vi "pyCode init.vi"(7 "pyCmdFilePath":path, 8 "error in (no error)":errorcluster, 10 "pyVersion":string, 11 "pyCode in":refnum<class "pyCode.lvclass">) -> (0 "error out":errorcluster, 3 "pyCode out":refnum<class "pyCode.lvclass">)   [LabVIEW 2018, in "pyCode.lvclass"]
uses:
  pyCode.lvclass
  pyCode.lvclass/pyCode.ctl
  Attributes/Write pyCmdFilePath.vi
  Attributes/Write pyCmdSession.vi
panel:
  out "standard output":string
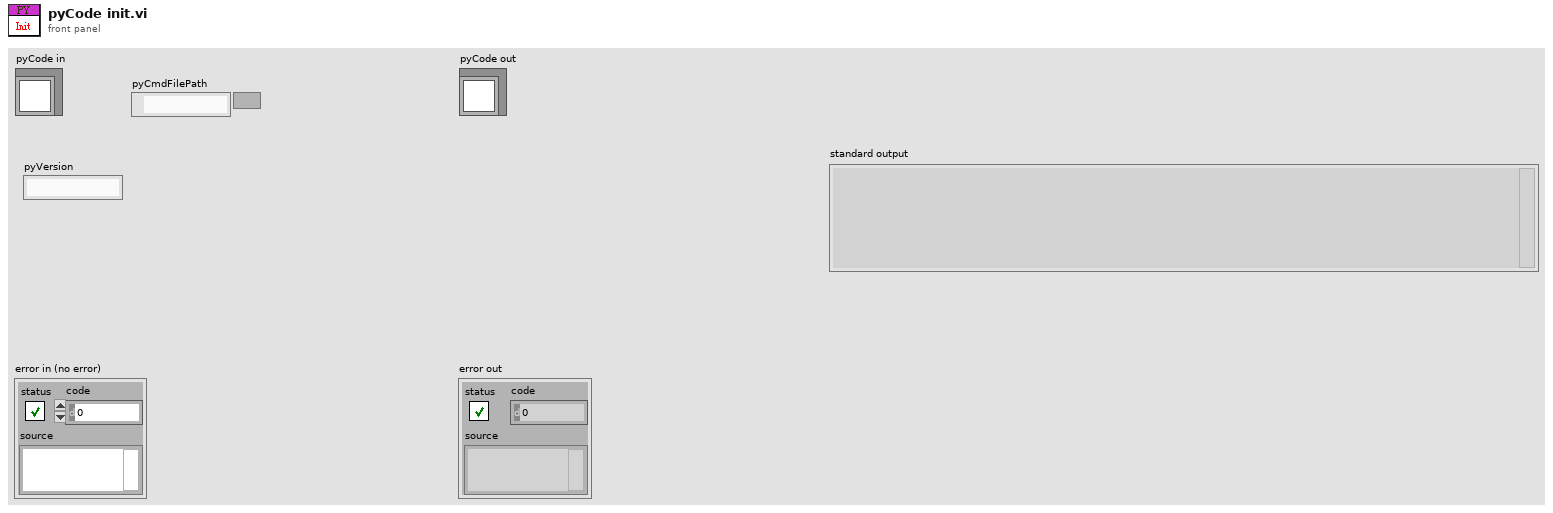
[diagram p1: front panel]
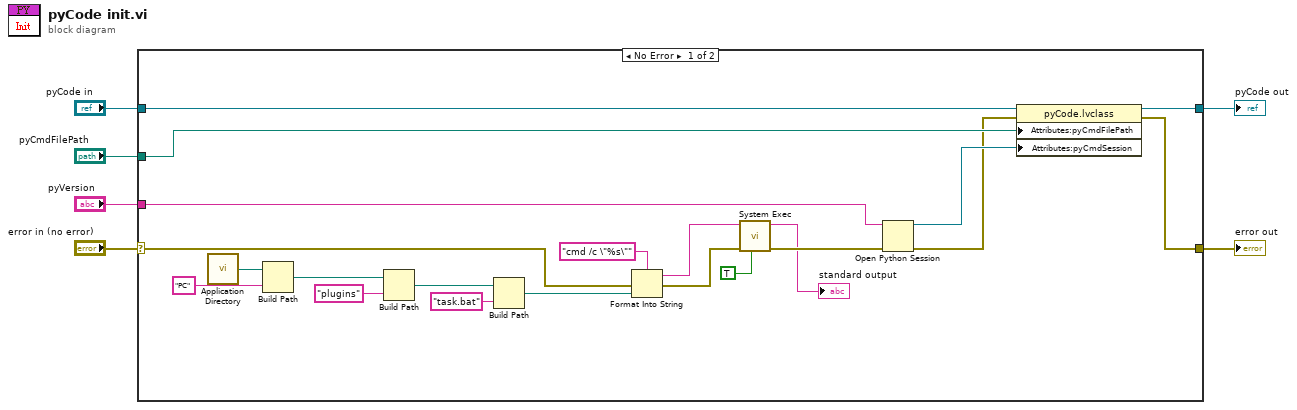
[diagram p0: block diagram]
diagram:
  n1 = case shown="No Error" "error in (no error)" {
    selector: "error in (no error)" -> [w10 w29]
    tunnel: [w21 w29] -> w5
    tunnel: [w26 w28] -> w3
    tunnel: "pyCode in" -> [w27 w28]
    tunnel: "pyVersion" -> [w25 _]
    tunnel: "pyCmdFilePath" -> [w23 _]
    frame No Error {
      n2 = call <vilib>:"Application Directory.vi"() -> ("Application Directory"=w19:path)
      n3 = Build Path(base path=w19, name or relative path="PC") -> (appended path=w18:path)
      n4 = Build Path(base path=w18, name or relative path="plugins") -> (appended path=w17:path)
      n5 = Build Path(base path=w17, name or relative path="task.bat") -> (appended path=w13:path)
      n6 = Format Into String(format string="cmd /c \"%s\"", error in=w10, w13) -> (resulting string=w12:string, error out=w9:errorcluster)  [unwired: 1 in]
      n7 = call <vilib>:"System Exec.vi"("run minimized? (F)"=TRUE, "error in (no error)"=w9, "command line"=w12) -> ("error out"=w8:errorcluster, "standard output"=→"standard output":string)  [unwired: 5 in, 2 out]
      n8 = Open Python Session(python version=w25, 3:w8) -> (session out=w24:refnum<k35>, error out=w22:errorcluster)  [unwired: 1 in]
      n9 = property class="pyCode.lvclass"(reference=w27, error in=w22, "Attributes:pyCmdFilePath"=w23, "Attributes:pyCmdSession"=w24) -> (reference out=w26:refnum<class "pyCode.lvclass">, error out=w21:errorcluster)
    }
    frame Error {
    }
  }
  "error out" <- w5
  "pyCode out" <- w3
